vi "Teleop Intake Control.vi"(1 "Manipulator Button Cluster":T2, 2 "Manipulator Axes":T1, 3 "Driver Axes":T1) -> ()   [LabVIEW 2015]
uses:
  Common Code/Gamepads/Button Cluster.ctl
  Common Code/Gamepads/Axes Cluster.ctl
  Common Code/Intake Commands.ctl
  Common Code/Change Detect.vi
  Common Code/Change Detect Boolean.vi
  Robot Global Data.vi
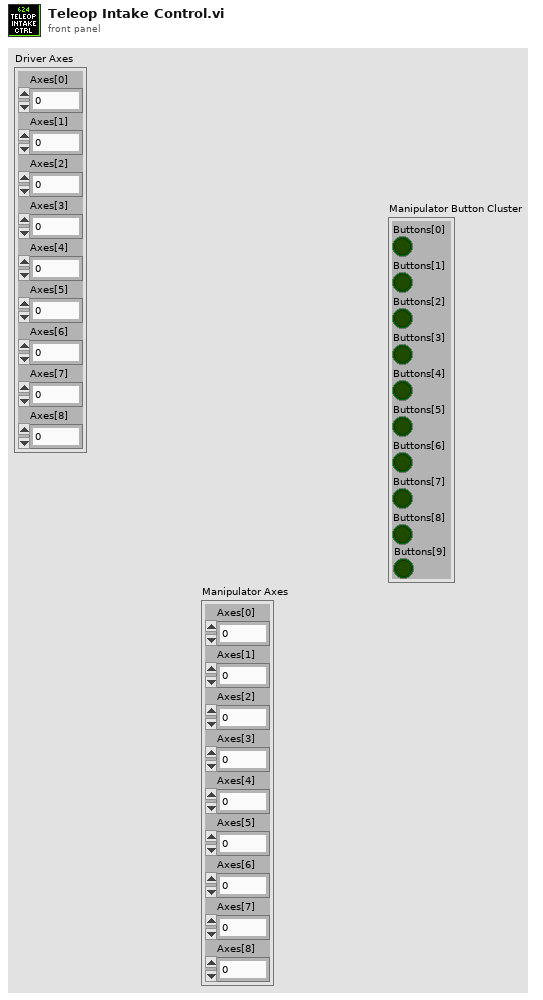
[diagram p1: front panel]
types:
  T1 = typedef "Axes Cluster.ctl" = cluster{"Axes[0]":dbl, "Axes[1]":dbl, "Axes[2]":dbl, "Axes[3]":dbl, "Axes[4]":dbl, "Axes[5]":dbl, "Axes[6]":dbl, "Axes[7]":dbl, "Axes[8]":dbl}
  T2 = typedef "Button Cluster.ctl" = cluster{"Buttons[0]":bool, "Buttons[1]":bool, "Buttons[2]":bool, "Buttons[3]":bool, "Buttons[4]":bool, "Buttons[5]":bool, "Buttons[6]":bool, "Buttons[7]":bool, "Buttons[8]":bool, "Buttons[9]":bool}
  T3 = typedef "Intake Commands.ctl" = enum16{"Settle Ball", "Unload", "Load", "Pull up", "Drop low", "Idle", "Lift Half", "Go To Angle"}
  T4 = enum16{"0", "1", "2", "3", "4", "5", "6", "7", "8", "9", "A", "B", "C", "D", "E", "F", "G", "H", "I", "J", "K", "L", "M", "N", "O", "P", "Q", "R", "S", "T", "U", "V", "W", "X", "Y", "Z", "F1", "F2", "F3", "F4", "F5", "F6", "F7", "F8", "F9", "F10", "F11", "F12", "F13", "F14", "F15", "ADD", "BACK", "BACKSLASH", "CAPITAL", "COMMA", "DECIMAL", "DELETE", "DIVIDE", "DOWN", "END", "EQUALS", "ESCAPE", "GRAVE (`)", "HOME", "INSERT", "LBRACKET", "LCONTROL", "LEFT", "L ALT", "LSHIFT", "LWIN", "MINUS", "MULTIPLY", "NEXT", "NUMLOCK", "NUMPAD_0", "NUMPAD_1", "NUMPAD_2", "NUMPAD_3", "NUMPAD_4", "NUMPAD_5", "NUMPAD_6", "NUMPAD_7", "NUMPAD_8", "NUMPAD_9", "PAUSE", "PERIOD", "PRIOR (PG UP)", "RBRACKET", "RCONTROL", "RETURN", "RIGHT", "R ALT", "RSHIFT", "RWIN", "SCROLL", "SEMICOLON", "SLASH", "SPACE", "SUBTRACT", "TAB", "UP", "ENTER (num pad)", "' (quote)"}
  T5 = typedef "Intake Mode.ctl" = enum16{"Safe", "Auto", "Manual"}
  T6 = typedef "Intake Commands Cluster.ctl" = cluster{"Intake Commands":T3, "Intake Mode":T5, "Override IR":bool, "Angle Target":dbl}
  T7 = typedef "Manual Intake Commands.ctl" = cluster{"Intake":bool, "Eject":bool, "Arm Angle":dbl, "Intake Override Speed":dbl, "Arm Override Speed":dbl, "Arm Speed":dbl, "Override Intake":bool, "Override Eject":bool, "Eject Override Speed":dbl, "Arm":bool, "Override Arm":bool, "Override Angle":bool}
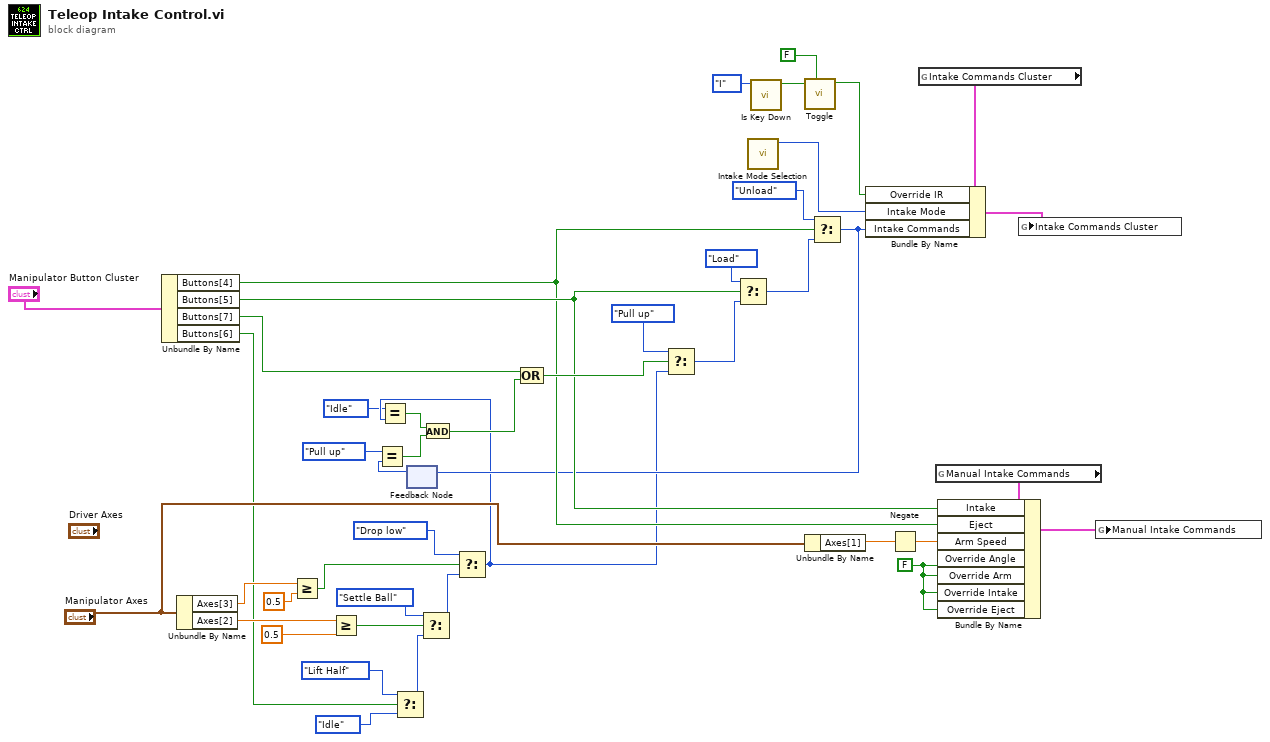
[diagram p0: block diagram]
diagram:
  w14 = FALSE ("Override Angle")
  n1 = Unbundle By Name("Manipulator Button Cluster") -> ("Buttons[4]"=w24:bool, "Buttons[5]"=w26:bool, "Buttons[7]"=w23:bool, "Buttons[6]"=w5:bool)
  n2 = Unbundle By Name("Manipulator Axes") -> ("Axes[3]"=w38:dbl, "Axes[2]"=w34:dbl)
  n3 = Greater Or Equal?(x=w38, y=0.5) -> (x >= y?=w25:bool)
  n4 = Greater Or Equal?(x=w34, y=0.5) -> (x >= y?=w3:bool)
  n5 = Select(t=Intake_Commands."Lift Half" ("f"), s=w5, f=Intake_Commands."Idle") -> (s? t:f=w4:T3)
  n6 = feedback #1() -> (w13:T3)  [unwired: 1 in]
  n7 = Equal?(x=Intake_Commands."Pull up", y=w13) -> (x = y?=w10:bool)
  n8 = Select(t=Intake_Commands."Settle Ball", s=w3, f=w4) -> (s? t:f=w1:T3)
  n9 = Select(t=Intake_Commands."Drop low" ("Intake Commands"), s=w25, f=w1) -> (s? t:f=w7:T3)
  n10 = Equal?(x=Intake_Commands."Idle", y=w7) -> (x = y?=w11:bool)
  n11 = And(x=w11, y=w10) -> (x .and. y?=w9:bool)
  n12 = Compound Arithmetic op=OR(w23, w9) -> (w30:bool)
  n13 = Select(t=Intake_Commands."Pull up" ("Intake Commands"), s=w30, f=w7) -> (s? t:f=w41:T3)
  n14 = Select(t=Intake_Commands."Load" ("Intake Commands"), s=w26, f=w41) -> (s? t:f=w32:T3)
  n15 = call "Intake Mode Selection.vi"() -> ("Mode"=w27:T5)  [unwired: 11 in]
  n16 = call "Is Key Down.vi"("Key"=T4."I") -> ("Key Down?"=w22:bool)  [unwired: 10 in]
  n17 = call "Toggle.vi"("Initial Value"=FALSE, "In"=w22) -> ("Toggled"=w16:bool)  [unwired: 9 in]
  n18 = Unbundle By Name("Manipulator Axes") -> ("Axes[1]"=w28:dbl)
  n19 = Select(t=Intake_Commands."Unload" ("Intake Commands"), s=w24, f=w32) -> (s? t:f=w12:T3)
  n20 = feedback-in #1(w12) -> ()
  n21 = Negate(x=w28) -> (-x=w19:dbl)
  n22 = global read "Robot Global Data.vi" "Intake Commands Cluster"() -> (w40:T6)
  n23 = Bundle By Name(cluster=w40, "Override IR"=w16, "Intake Mode"=w27, "Intake Commands"=w12) -> (w39:T6)
  n24 = global read "Robot Global Data.vi" "Manual Intake Commands"() -> (w18:T7)
  n25 = Bundle By Name(cluster=w18, "Intake"=w26, "Eject"=w24, "Arm Speed"=w19, "Override Angle"=w14, "Override Arm"=w14, "Override Intake"=w14, "Override Eject"=w14) -> (w20:T7)
  n26 = global write "Robot Global Data.vi" "Intake Commands Cluster"(w39) -> ()
  n27 = global write "Robot Global Data.vi" "Manual Intake Commands"(w20) -> ()
